vi "Custom source-meter - Disconnect.vi"(8 "Error In":errorcluster, 11 "Source-meter handle in":T1) -> (0 "Error Out":errorcluster, 3 "Source-meter handle out":T1)   [LabVIEW 2019]
doc: "This subVI is meant to perform all operations necessary to terminate the connection with your source meter. Source-meter handle parameters, including your custom settings are made available to you. Remember to return connection status to the Source-meter handle indicator."
uses:
  Type defs/Source-meter handle Type Def.ctl
  Type defs/Source-meter Type Def.ctl
  Custom source-meter settings.ctl
panel:
  # "Place all operations necessary to disconnect your custom source-meter in this VI"
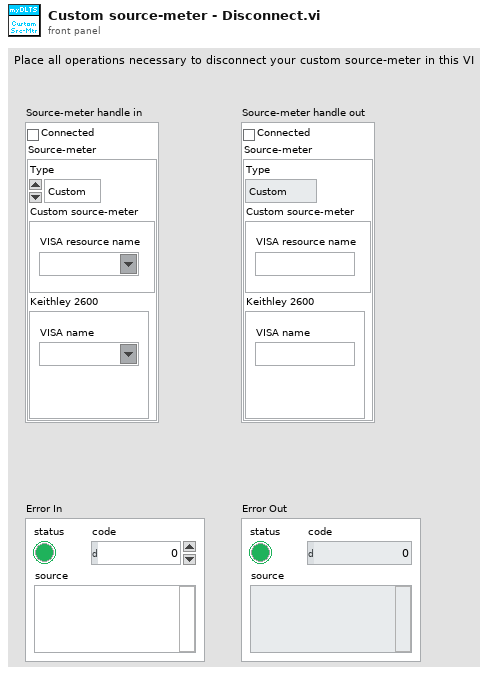
[diagram p1: front panel]
types:
  T1 = typedef "Source-meter handle Type Def.ctl" = cluster{"Connected":bool, "Source-meter":T2}
  T2 = typedef "Source-meter Type Def.ctl" = cluster{"Type":enum16{"Custom", "Keithley 2600"}, "Custom source-meter":T3, "Keithley 2600":cluster{"VISA name":refnum<visa-resource-name>}}
  T3 = typedef "Custom source-meter settings.ctl" = cluster{"VISA resource name":refnum<visa-resource-name>}
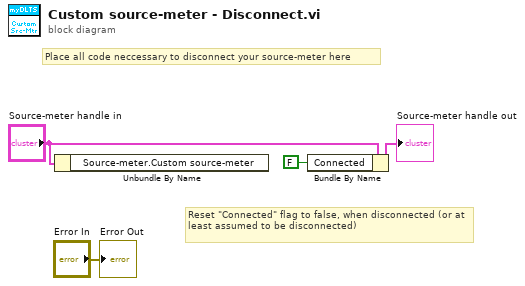
[diagram p0: block diagram]
diagram:
  # "Reset \"Connected\" flag to false, when disconnected (or at least assumed to be disconnected)"
  # "Place all code neccessary to disconnect your source-meter here"
  n1 = Unbundle By Name("Source-meter handle in") -> ()  [unwired: 1 out]
  n2 = Bundle By Name(cluster="Source-meter handle in", "Connected"=FALSE) -> (→"Source-meter handle out":T1)
  "Error Out" <- "Error In"
